vi "CONFIGURE_DIGITIZER_1.vi"(5 "TRIGGER SETTINGS IN":T2, 6 "error in":errorcluster, 7 "Horizontal Settings IN":T1, 8 "Vertical Settings IN":T3, 9 "DIGITIZER 1 CHANNELS":string) -> (0 "error out":errorcluster, 1 "TRIGGER SETTINGS OUT":T2, 2 "Gain Multiplier":dbl, 3 "instrument handle out":refnum<k15>, 4 "VERTICAL SETTINGS OUT":T3)   [LabVIEW 2010]
uses:
  <instrlib>/niScope/Controls/niScope trigger slope.ctl
  <instrlib>/niScope/Controls/niScope trigger source.ctl
  <instrlib>/niScope/Controls/niScope export destinations.ctl
  <instrlib>/niScope/Controls/niScope exportable signals.ctl
  <instrlib>/niScope/Controls/niScope trigger source digital.ctl
  <instrlib>/niScope/Configure/Trigger/niScope Configure Trigger Edge.vi
  <instrlib>/niScope/Configure/Trigger/niScope Configure Trigger Digital.vi
  <instrlib>/niScope/Configure/Trigger/niScope Configure Trigger Immediate.vi
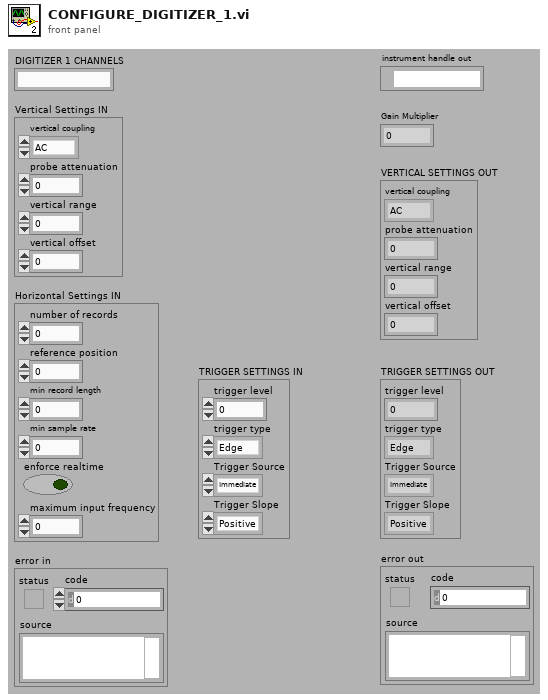
[diagram p1: front panel]
types:
  T1 = cluster{"number of records":i32, "reference position":dbl, "min record length":i32, "min sample rate":dbl, "enforce realtime":bool, "maximum input frequency":dbl}
  T2 = cluster{"trigger level":dbl, "trigger type":enum16{"Edge", "Digital", "Immediate"}, "Trigger Source":enum8{"Immediate", "Channel 0", "Channel 1", "Channel 2", "Channel 3", "Channel 4", "Channel 5", "Channel 6", "Channel 7", "External TRIG", "Software Trigger", "RTSI 0", "RTSI 1", "RTSI 2", "RTSI 3", "RTSI 4", "RTSI 5", "RTSI 6", "PFI 0", "PFI 1", "PFI 2", "PXI Star Trigger"}, "Trigger Slope":enum16{"Positive", "Negative"}}
  T3 = cluster{"vertical coupling":enum16{"AC", "DC", "Ground"}, "probe attenuation":dbl, "vertical range":dbl, "vertical offset":dbl}
  T4 = enum8{"Immediate", "Channel 0", "Channel 1", "Channel 2", "Channel 3", "Channel 4", "Channel 5", "Channel 6", "Channel 7", "External TRIG", "Software Trigger", "RTSI 0", "RTSI 1", "RTSI 2", "RTSI 3", "RTSI 4", "RTSI 5", "RTSI 6", "PFI 0", "PFI 1", "PFI 2", "PXI Star Trigger"}
  T5 = typedef "niScope trigger source.ctl" = string
  T6 = typedef "niScope export destinations.ctl" = string
  T7 = typedef "niScope trigger source digital.ctl" = string
  T8 = typedef "niScope trigger slope.ctl" = i32
  T9 = typedef "niScope exportable signals.ctl" = u16
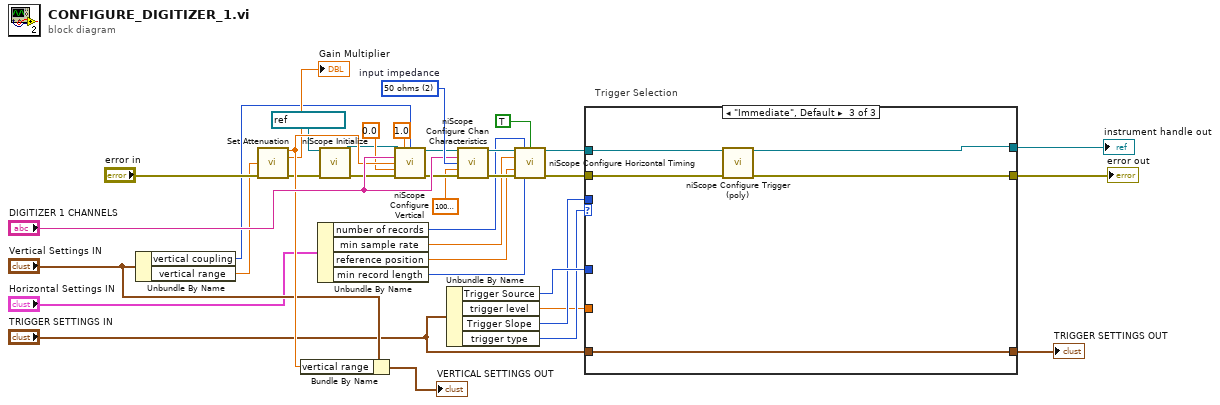
[diagram p0: block diagram]
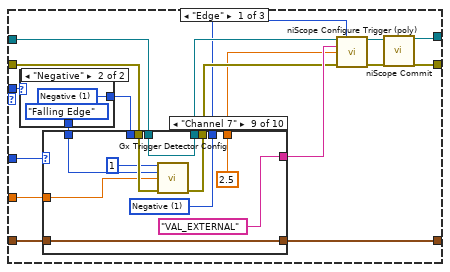
[diagram p2: hidden frame]
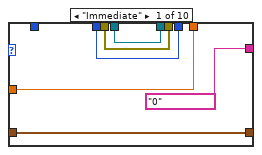
[diagram p3: hidden frame]
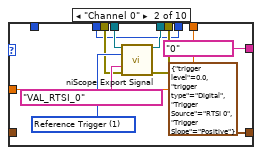
[diagram p4: hidden frame]
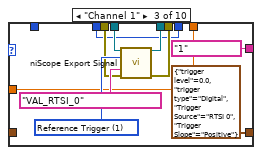
[diagram p5: hidden frame]
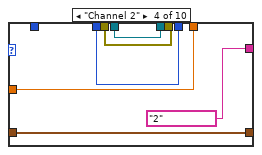
[diagram p6: hidden frame]
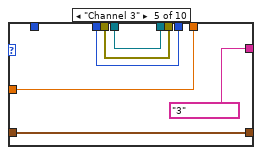
[diagram p7: hidden frame]
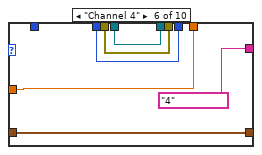
[diagram p8: hidden frame]
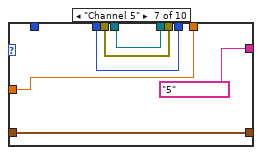
[diagram p9: hidden frame]
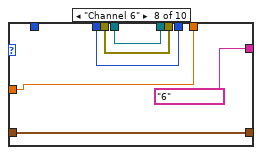
[diagram p10: hidden frame]
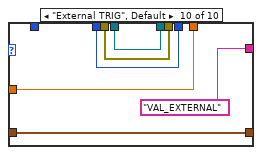
[diagram p11: hidden frame]
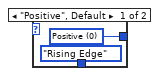
[diagram p12: hidden frame]
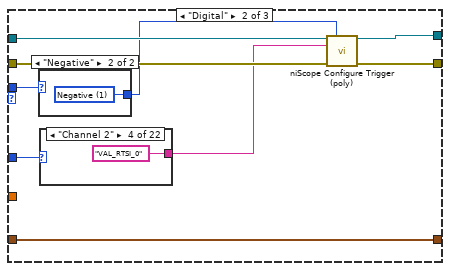
[diagram p13: hidden frame]
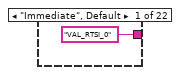
[diagram p14: hidden frame]
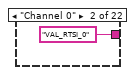
[diagram p15: hidden frame]
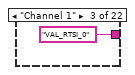
[diagram p16: hidden frame]
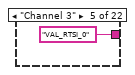
[diagram p17: hidden frame]
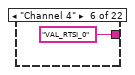
[diagram p18: hidden frame]
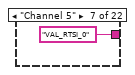
[diagram p19: hidden frame]
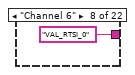
[diagram p20: hidden frame]
diagram:
  w36 = u32 2 items=["1 mega ohm"=0, "50 ohms"=2]  # input impedance
  n1 = Unbundle By Name("Vertical Settings IN") -> ("vertical coupling"=w8:enum16{"AC", "DC", "Ground"}, "vertical range"=w10:dbl)
  n2 = call "Set Attenuation.vi"("vertical range"=w10, "error in"="error in") -> ("Requested Range"=w30:dbl, "Gain Multiplier"=→"Gain Multiplier":dbl, "error out"=w12:errorcluster)  [unwired: 11 in]
  n3 = Bundle By Name(cluster="Vertical Settings IN", "vertical range"=w30) -> (→"VERTICAL SETTINGS OUT":T3)
  n4 = Unbundle By Name("Horizontal Settings IN") -> ("number of records"=w16:i32, "min sample rate"=w17:dbl, "reference position"=w18:dbl, "min record length"=w19:i32)
  n5 = call <instrlib>:"niScope Initialize.vi"("resource name"=refnum<k15> "PXI1Slot6", "error in"=w12) -> ("instrument handle"=w2:refnum<k15>, "error out"=w5:errorcluster)  [unwired: 12 in]
  n6 = call <instrlib>:"niScope Configure Vertical.vi"("instrument handle"=w2, "probe attenuation"=1.0, "vertical coupling"=w8, "channels"="DIGITIZER 1 CHANNELS", "vertical range"=w30, "vertical offset"=0.0, "error in"=w5) -> ("instrument handle out"=w33:refnum<k15>, "error out"=w14:errorcluster)  [unwired: 7 in]
  n7 = Unbundle By Name("TRIGGER SETTINGS IN") -> ("Trigger Source"=w26:T4, "trigger level"=w20:dbl, "Trigger Slope"=w25:enum16{"Positive", "Negative"}, "trigger type"=w24:enum16{"Edge", "Digital", "Immediate"})
  n8 = call <instrlib>:"niScope Configure Chan Characteristics.vi"("instrument handle"=w33, "channels"="DIGITIZER 1 CHANNELS", "input impedance"=w36, "maximum input frequency"=10000000.0, "error in"=w14) -> ("instrument handle out"=w34:refnum<k15>, "error out"=w32:errorcluster)  [unwired: 9 in]
  n9 = call <instrlib>:"niScope Configure Horizontal Timing.vi"("instrument handle"=w34, "number of records"=w16, "enforce realtime"=TRUE, "min sample rate"=w17, "reference position"=w18, "error in"=w32, "min record length"=w19) -> ("instrument handle out"=w4:refnum<k15>, "error out"=w3:errorcluster)  [unwired: 7 in]
  n10 = case "Trigger Selection" shown="\"Immediate\", Default" w24 {
    tunnel: w3 -> [w43 w139 w168]
    tunnel: [w48 w132 w165] -> w6
    tunnel: w4 -> [w45 w138 w167]
    tunnel: [w49 w133 w166] -> w21
    tunnel: w26 -> [w53 w135 _]
    tunnel: w20 -> [w39 _ _]
    tunnel: w25 -> [w54 w137 _]
    tunnel: "TRIGGER SETTINGS IN" -> [w47 w131 w164]
    tunnel: [w46 w131 w164] -> w28
    frame "Edge" {
      n11 = case shown="\"Negative\"" w54 {
        tunnel: [w128 w130] -> w41
        tunnel: [enum16{"Rising Edge", "Falling Edge"}."Rising Edge" ("Slope") enum16{"Rising Edge", "Falling Edge"}."Falling Edge" ("Slope")] -> w37
        frame "Positive", Default {
          w128 = T8 0 items=["Positive", "Negative"] ("trigger slope")
        }
        frame "Negative" {
          w130 = T8 1 items=["Positive", "Negative"] ("trigger slope")
        }
      }
      n12 = case shown="\"Channel 7\"" w53 {
        tunnel: [T5 "0" ("trigger source") T5 "0" ("trigger source") T5 "1" ("trigger source") T5 "2" ("trigger source") T5 "3" ("trigger source") T5 "4" ("trigger source") T5 "5" ("trigger source") T5 "6" ("trigger source") T5 "VAL_EXTERNAL" ("trigger source") T5 "VAL_EXTERNAL" ("trigger source")] -> w52
        tunnel: w47 -> [w59 _ _ w85 w91 w97 w103 w109 w119 w125]
        tunnel: [w59 T2 {"trigger level"=0.0, "trigger type"=enum."Digital", "Trigger Source"=enum."RTSI 0", "Trigger Slope"=enum."Positive"} ("Trigger settings") T2 {"trigger level"=0.0, "trigger type"=enum."Digital", "Trigger Source"=enum."RTSI 0", "Trigger Slope"=enum."Positive"} ("Trigger settings") w85 w91 w97 w103 w109 w119 w125] -> w46
        tunnel: w45 -> [w58 w66 w76 w84 w90 w96 w102 w108 w118 w124]
        tunnel: [w58 w64 w75 w84 w90 w96 w102 w108 w118 w124] -> w44
        tunnel: w43 -> [w57 w65 w74 w83 w89 w95 w101 w107 w115 w123]
        tunnel: [w57 w63 w73 w83 w89 w95 w101 w107 w114 w123] -> w42
        tunnel: w41 -> [w56 w62 w72 w82 w88 w94 w100 w106 _ w122]
        tunnel: [w56 w62 w72 w82 w88 w94 w100 w106 w116 w122] -> w40
        tunnel: [w55 w61 w71 w81 w87 w93 w99 w105 2.5 ("trigger level") w121] -> w38
        tunnel: w39 -> [w55 w61 w71 w81 w87 w93 w99 w105 w112 w121]
        tunnel: w37 -> [_ _ _ _ _ _ _ _ w111 _]
        frame "Immediate" {
        }
        frame "Channel 0" {
          w67 = T9 1 items=["None"=0, "Start Trigger"=2, "Advance Trigger"=5, "Reference Trigger"=1, "End of Record Event"=4, "End of Acquisition Event"=3, "Ready for Start Event"=7, "Ready for Advance Event"=6, "Ready for Reference Event"=10, "Reference Clock"=100, "Sample Clock"=101, "5 Volt Power"=13] ("signal")
          n13 = call <instrlib>:"niScope Export Signal.vi"("instrument handle"=w66, "signal"=w67, "output terminal"=T6 "VAL_RTSI_0", "error in"=w65) -> ("instrument handle out"=w64:refnum<k15>, "error out"=w63:errorcluster)  [unwired: 10 in]
        }
        frame "Channel 1" {
          w77 = T9 1 items=["None"=0, "Start Trigger"=2, "Advance Trigger"=5, "Reference Trigger"=1, "End of Record Event"=4, "End of Acquisition Event"=3, "Ready for Start Event"=7, "Ready for Advance Event"=6, "Ready for Reference Event"=10, "Reference Clock"=100, "Sample Clock"=101, "5 Volt Power"=13] ("signal")
          n14 = call <instrlib>:"niScope Export Signal.vi"("instrument handle"=w76, "signal"=w77, "output terminal"=T6 "VAL_RTSI_0", "error in"=w74) -> ("instrument handle out"=w75:refnum<k15>, "error out"=w73:errorcluster)  [unwired: 10 in]
        }
        frame "Channel 2" {
        }
        frame "Channel 3" {
        }
        frame "Channel 4" {
        }
        frame "Channel 5" {
        }
        frame "Channel 6" {
        }
        frame "Channel 7" {
          w116 = T8 1 items=["Positive", "Negative"] ("trigger slope")
          n15 = call "Gx Trigger Detector Config.vi"("Slot"=i16 1, "Slope"=w111, "Trigger Voltage"=w112, "error in (no error)"=w115) -> ("error out"=w114:errorcluster)  [unwired: 10 in, 1 out]
        }
        frame "External TRIG", Default {
        }
      }
      n16 = call-poly <instrlib>:"niScope Configure Trigger (poly).vi"("instrument handle"=w44, "trigger slope"=w40, "trigger source"=w52, "trigger level"=w38, "error in"=w42) -> ("instrument handle out"=w51:refnum<k15>, "error out"=w50:errorcluster)  [unwired: 9 in]
      n17 = call <instrlib>:"niScope Commit.vi"("instrument handle"=w51, "error in"=w50) -> ("instrument handle out"=w49:refnum<k15>, "error out"=w48:errorcluster)  [unwired: 12 in]
    }
    frame "Digital" {
      n18 = case shown="\"Negative\"" w137 {
        tunnel: [w162 w163] -> w136
        frame "Positive", Default {
          w162 = T8 0 items=["Positive", "Negative"] ("trigger slope")
        }
        frame "Negative" {
          w163 = T8 1 items=["Positive", "Negative"] ("trigger slope")
        }
      }
      n19 = case shown="\"Channel 2\"" w135 {
        tunnel: [T7 "VAL_RTSI_0" ("trigger source") T7 "VAL_RTSI_0" ("trigger source") T7 "VAL_RTSI_0" ("trigger source") T7 "VAL_RTSI_0" ("trigger source") T7 "VAL_RTSI_0" ("trigger source") T7 "VAL_RTSI_0" ("trigger source") T7 "VAL_RTSI_0" ("trigger source") T7 "VAL_RTSI_0" ("trigger source") T7 "VAL_RTSI_0" ("trigger source") T7 "VAL_RTSI_0" ("trigger source") T7 "VAL_RTSI_0" ("trigger source") T7 "VAL_RTSI_0" ("trigger source") T7 "VAL_RTSI_1" ("trigger source") T7 "VAL_RTSI_2" ("trigger source") T7 "VAL_RTSI_3" ("trigger source") T7 "VAL_RTSI_4" ("trigger source") T7 "VAL_RTSI_5" ("trigger source") T7 "VAL_RTSI_6" ("trigger source") T7 "VAL_PFI_0" ("trigger source") T7 "VAL_PFI_1" ("trigger source") T7 "VAL_PFI_2" ("trigger source") T7 "VAL_PXI_STAR" ("trigger source")] -> w134
        frame "Immediate", Default {
        }
        frame "Channel 0" {
        }
        frame "Channel 1" {
        }
        frame "Channel 2" {
        }
        frame "Channel 3" {
        }
        frame "Channel 4" {
        }
        frame "Channel 5" {
        }
        frame "Channel 6" {
        }
        frame "Channel 7" {
        }
        frame "External TRIG" {
        }
        frame "Software Trigger" {
        }
        frame "RTSI 0" {
        }
        frame "RTSI 1" {
        }
        frame "RTSI 2" {
        }
        frame "RTSI 3" {
        }
        frame "RTSI 4" {
        }
        frame "RTSI 5" {
        }
        frame "RTSI 6" {
        }
        frame "PFI 0" {
        }
        frame "PFI 1" {
        }
        frame "PFI 2" {
        }
        frame "PXI Star Trigger" {
        }
      }
      n20 = call-poly <instrlib>:"niScope Configure Trigger (poly).vi"("instrument handle"=w138, "trigger slope"=w136, "trigger source"=w134, "error in"=w139) -> ("instrument handle out"=w133:refnum<k15>, "error out"=w132:errorcluster)  [unwired: 10 in]
    }
    frame "Immediate", Default {
      n21 = call-poly <instrlib>:"niScope Configure Trigger (poly).vi"("instrument handle"=w167, "error in"=w168) -> ("instrument handle out"=w166:refnum<k15>, "error out"=w165:errorcluster)  [unwired: 12 in]
    }
  }
  "TRIGGER SETTINGS OUT" <- w28
  "instrument handle out" <- w21
  "error out" <- w6
